vi "Complex LU Factorization.vi"(0 "A":T1) -> (1 "L":T1, 2 "U":T1, 3 "P":i32[][](array[numeric]), 4 "error":i32)   [LabVIEW 2024, in "NI_AALPro.lvlib"]
doc: "<p>Performs the LU factorization of <strong>A</strong> so that <strong>PA</strong> = <strong>LU</strong>. Wire data to the <strong>A</strong> input to determine the polymorphic instance to use or <a href=\"nihelplauncher://docs/csh?context=lvcore_lvhowto_selectingdefaultinstpolyvi\">manually select</a> the instance.</p>"
uses:
  NI_AALPro.lvlib
  ComplexMatrix.ctl
  NI_AALBase.lvlib
  NI_Matrix.lvlib
panel:
  # "Complex LU Factorization"
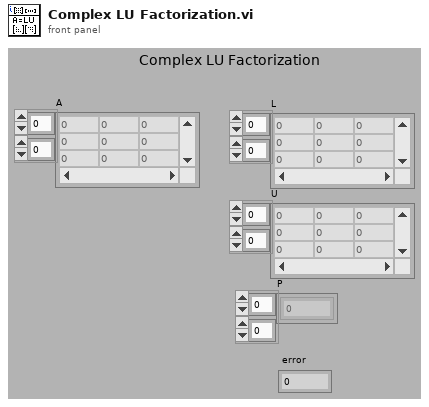
[diagram p1: front panel]
types:
  T1 = typedef "NI_Matrix.lvlib/ComplexMatrix.ctl" = cdb[][]
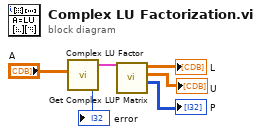
[diagram p0: block diagram]
diagram:
  n1 = call "Complex LU Factor.vi"("A"="A") -> ("LU Info"=w1:cluster{"LU":cdb[][], "Pivot":i32[]}, "error"=→"error":i32)  [unwired: 1 out]
  n2 = call "Get Complex LUP Matrix.vi"("LU Info"=w1) -> ("L"=→"L":T1, "U"=→"U":T1, "P"=→"P":i32[][])  [unwired: 1 in]
